vi "Write.vi"(6 "Append Index":i32, 8 "error in (no error)":errorcluster, 9 "Notes":string, 10 "Data (Dictionary)":T1[](array[typedef]), 11 "Data.DAT in":refnum<class "Data.DAT.lvclass">) -> (0 "error out":errorcluster, 3 "Data.DAT out":refnum<class "Data.DAT.lvclass">, 5 "Path out":path)   [LabVIEW 2019, in "Data.DAT.lvclass"]
uses:
  Data.DAT.lvclass
  Data/Data.lvclass
  C:/Program Files (x86)/National Instruments/LabVIEW 2020/user.lib/LevyLab/LV to ITX/Data/Data.lvclass
  Write DAT (2D).vi
  Data/Typedefs/Dictionary--cluster.ctl
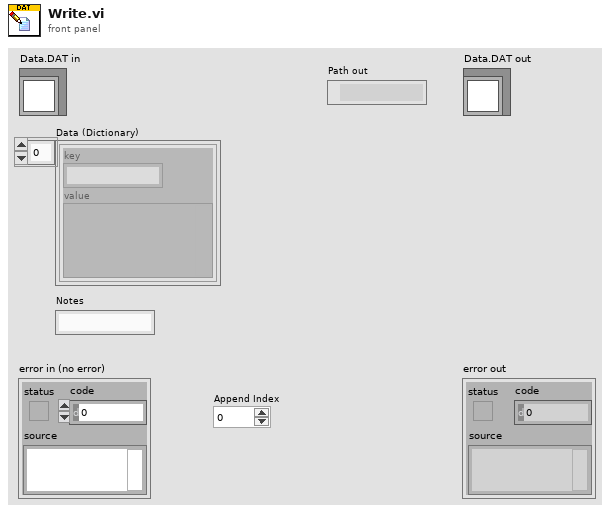
[diagram p1: front panel]
types:
  T1 = typedef "Data.lvclass/Dictionary--cluster.ctl" = cluster{"key":string, "value":variant}
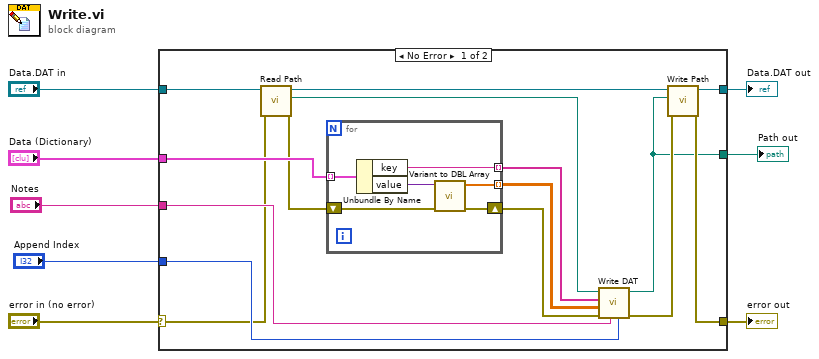
[diagram p0: block diagram]
diagram:
  n1 = case shown="No Error" "error in (no error)" {
    selector: "error in (no error)" -> [w9 w31]
    tunnel: [w21 w31] -> w7
    tunnel: "Data.DAT in" -> [w12 w30]
    tunnel: [w23 w30] -> w5
    tunnel: "Data (Dictionary)" -> [w16 _]
    tunnel: "Notes" -> [w13 _]
    tunnel: [w11 _] -> w2
    tunnel: "Append Index" -> [w10 _]
    frame No Error {
      n2 = call "Read Path.vi"("error in (no error)"=w9, "Data Save"=w12) -> ("error out"=w14:errorcluster, "Path"=w15:path, "Data Save out"=w18:refnum<class "Data.DAT.lvclass">)  [unwired: 7 in]
      n3 = for {
        tunnel: w16 -> [w29] mode=indexing
        tunnel: [w28] -> w19 mode=indexing
        tunnel: [w26] -> w17 mode=indexing
        shift-right: [w24] -> w20
        shift-left: w14 -> [w25]
        n4 = Unbundle By Name(w29) -> ("key"=w28:string, "value"=w27:variant)
        n5 = call "Variant to DBL Array.vi"("error in (no error)"=w25, "Data (Variant)"=w27) -> ("error out"=w24:errorcluster, "1D Array"=w26:dbl[])  [unwired: 7 in, 1 out]
      }
      n6 = call-poly "Write DAT.vi"("Append (0=F)"=w10, "Comments"=w13, "error in"=w20, "Data"=w17, "Headers"=w19, "path"=w15) -> ("error out"=w22:errorcluster, "new file path"=w11:path)  [unwired: 4 in]
      n7 = call "Write Path.vi"("error in (no error)"=w22, "Path"=w11, "Data Save"=w18) -> ("error out"=w21:errorcluster, "Data Save out"=w23:refnum<class "Data.DAT.lvclass">)  [unwired: 7 in]
    }
    frame Error {
    }
  }
  "error out" <- w7
  "Data.DAT out" <- w5
  "Path out" <- w2
